vi "Tell.vi"(4 "Priority":bool, 10 "Msg":refnum<class "Msg.lvclass">, 11 "Event Transport in":refnum<class "Event Transport.lvclass">) -> (0 "Error out":errorcluster)   [LabVIEW 2025, in "jettl.lvlib" / "Transport.lvlib" / "Event Transport.lvclass"]
uses:
  Event Transport.lvclass
  Msg/Msg.lvclass
  Event Transport.lvclass/Event Transport.ctl
  <vilib>/event_ctls.llb/usereventprio.ctl
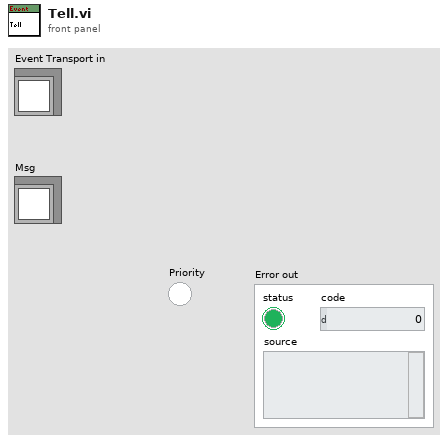
[diagram p1: front panel]
types:
  T1 = typedef "usereventprio.ctl" = enum32{"high priority", "normal priority"}
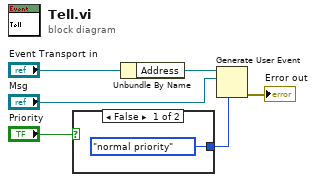
[diagram p0: block diagram]
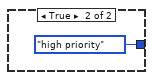
[diagram p2: hidden frame]
diagram:
  n1 = case shown="False" "Priority" {
    tunnel: [usereventprio."normal priority" ("priority (normal)") usereventprio."high priority" ("priority (normal)")] -> w1
    frame False {
    }
    frame True {
    }
  }
  n2 = Unbundle By Name("Event Transport in") -> ("Address"=w5:refnum<user-event>)
  n3 = Generate User Event(priority (normal)=w1, user event=w5, event data cluster="Msg") -> (error out=→"Error out":errorcluster)  [unwired: 1 in, 1 out]
